vi "destroy.vi"(8 "error in (no error)":errorcluster, 11 "system.threading in":refnum<class "system.threading.lvclass">) -> (0 "error out":errorcluster)   [LabVIEW 2021, in "system.threading.lvclass"]
uses:
  system.threading.lvclass
  system.threading.lvclass/system.threading.ctl
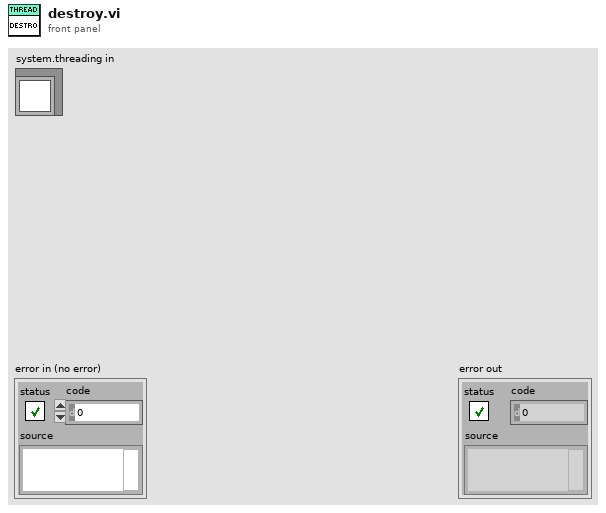
[diagram p1: front panel]
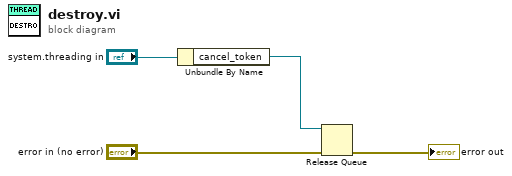
[diagram p0: block diagram]
diagram:
  n1 = Unbundle By Name("system.threading in") -> ("cancel_token"=w3:refnum<queue>)
  n2 = Release Queue(queue=w3, error in (no error)="error in (no error)") -> (error out=→"error out":errorcluster)  [unwired: 1 in, 2 out]
